vi "OP300ZP_Param_ConfZENplusOP100.vi"(8 "errin":errorcluster, 10 "Chaîne":string, 11 "pathin":path) -> (0 "errout":errorcluster, 3 "VISA OUT":T1)   [LabVIEW 2020]
uses:
  <vilib>/Utility/config.llb/Read Key (String).vi
  <vilib>/Utility/config.llb/NI_LVConfig.lvlib
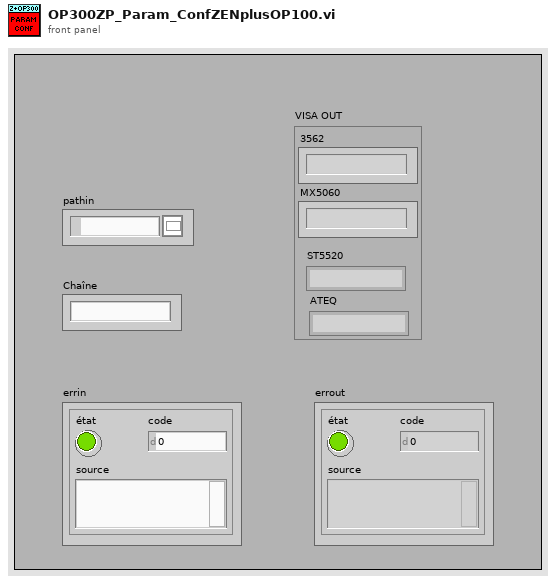
[diagram p1: front panel]
types:
  T1 = cluster{"3562":string, "MX5060":string, "ST5520":string, "ATEQ":string}
  T2 = typedef "NI_LVConfig.lvlib/Config Data RefNum.ctl" = refnum<k1>
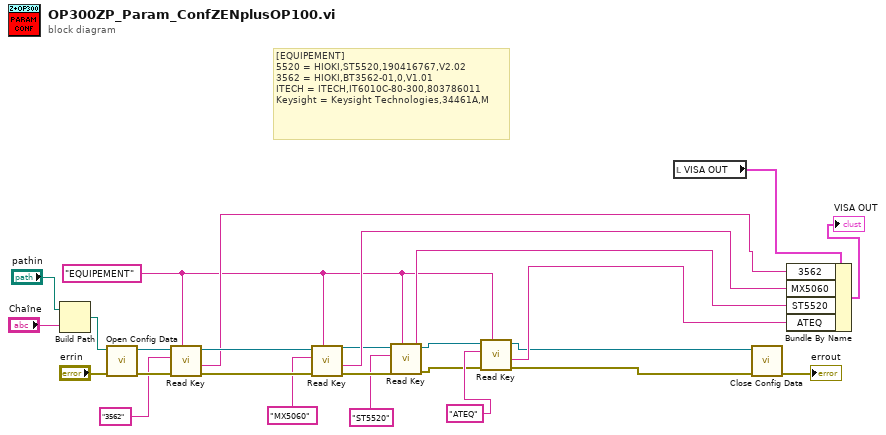
[diagram p0: block diagram]
diagram:
  w5 = "EQUIPEMENT" ("section")
  # "[EQUIPEMENT]\n5520 = HIOKI,ST5520,190416767,V2.02\n3562 = HIOKI,BT3562-01,0,V1.01\nITECH = ITECH,IT6010C-80-300,803786011\nKeysight = Keysight Technologies,34461A,M"
  n1 = Build Path(base path="pathin", name or relative path="Chaîne") -> (appended path=w23:path)
  n2 = call <vilib>:"Open Config Data.vi"("error in (no error)"="errin", "configuration file path"=w23) -> ("error out"=w25:errorcluster, "refnum"=w26:T2)  [unwired: 7 in, 1 out]
  n3 = call-poly <vilib>:"Read Key.vi"("section"=w5, "error in (no error)"=w25, "key"="3562", "refnum"=w26) -> ("error out"=w20:errorcluster, "value"=w15:string, "refnum out"=w22:T2)  [unwired: 4 in, 1 out]
  n4 = call-poly <vilib>:"Read Key.vi"("section"=w5, "error in (no error)"=w20, "key"="MX5060", "refnum"=w22) -> ("error out"=w10:errorcluster, "value"=w14:string, "refnum out"=w9:T2)  [unwired: 4 in, 1 out]
  n5 = call-poly <vilib>:"Read Key.vi"("section"=w5, "error in (no error)"=w10, "key"="ST5520", "refnum"=w9) -> ("error out"=w4:errorcluster, "value"=w13:string, "refnum out"=w2:T2)  [unwired: 4 in, 1 out]
  n6 = call-poly <vilib>:"Read Key.vi"("section"=w5, "error in (no error)"=w4, "key"="ATEQ", "refnum"=w2) -> ("error out"=w3:errorcluster, "value"=w7:string, "refnum out"=w1:T2)  [unwired: 4 in, 1 out]
  n7 = local read "VISA OUT"() -> (w16:T1)
  n8 = call <vilib>:"Close Config Data.vi"("error in (no error)"=w3, "refnum"=w1) -> ("error out"=→"errout":errorcluster)  [unwired: 8 in, 1 out]
  n9 = Bundle By Name(cluster=w16, "3562"=w15, "MX5060"=w14, "ST5520"=w13, "ATEQ"=w7) -> (→"VISA OUT":T1)
